vi "MyTestSimple.vi"() -> ()   [LabVIEW 2018]
uses:
  VisionLibrariesXimea/xiLib/xiLIB_64bit/xiLIB/xiCamLib/xiCam/PRM/PRM/PRM_v2.ctl
  VisionLibrariesXimea/xiLib/xiLIB_64bit/xiLIB/xiCamLib/xiLIB/Typedefs/xiLIB - PRM_Type.ctl
  D:/codes labview/VisionLibrariesXimea/xiLib/xiLIB_64bit/xiLIB/xiCamLib/API/x64/xiApi.NETX64.dll
  VisionLibrariesXimea/xiLib/xiLIB_64bit/xiLIB/xiCamLib/API/x64/xiApi.NETX64.dll
  <vilib>/Platform/TimedLoop/XDataNode/timing_clust.ctl
  <vilib>/Platform/TimedLoop/XDataNode/nitl_modes.ctl
  <vilib>/Platform/TimedLoop/XDataNode/wakeup.ctl
  System.Drawing
  VisionLibrariesXimea/xiLib/xiLIB_64bit/xiLIB/xiCamLib/xiLIB/xiLIB - GetPRM_INFO.vi
  VisionLibrariesXimea/xiLib/xiLIB_64bit/xiLIB/xiCamLib/xiCam/Methods/xiCam - GetParam_Int32.vi
  VisionLibrariesXimea/xiLib/xiLIB_64bit/xiLIB/xiCamLib/xiCam/Methods/xiCam - GetParam_Float.vi
  VisionLibrariesXimea/xiLib/xiLIB_64bit/xiLIB/xiCamLib/xiCam/Methods/xiCam - GetParam_String.vi
  <vilib>/platform/TimedLoop/XDataNode/XDataNode.xnode
  <vilib>/Platform/TimedLoop/XDataNode/XDNodeRunTimeDep.lvlib
panel:
  in  "Tab Control":T1(tab)
  in  "get float":T2
  out "output":variant
  out "Type":T3
  out "Desc.":string
  in  "start single":bool
  out "Waveform Graph 2":u8[](graph)
  out "Intensity Graph":u8[][](graph)
  in  "start loop acquire":bool
  out "Waveform Graph":u8[](graph)
  out "Numeric":i32
  out "Image":T4(plugin-control)
  in  "start NET":bool
  out "Numeric 2":i32
  in  "clear error":bool
  in  "dimension size":i32=16106496
  out "error out":errorcluster
  in  "stop":bool
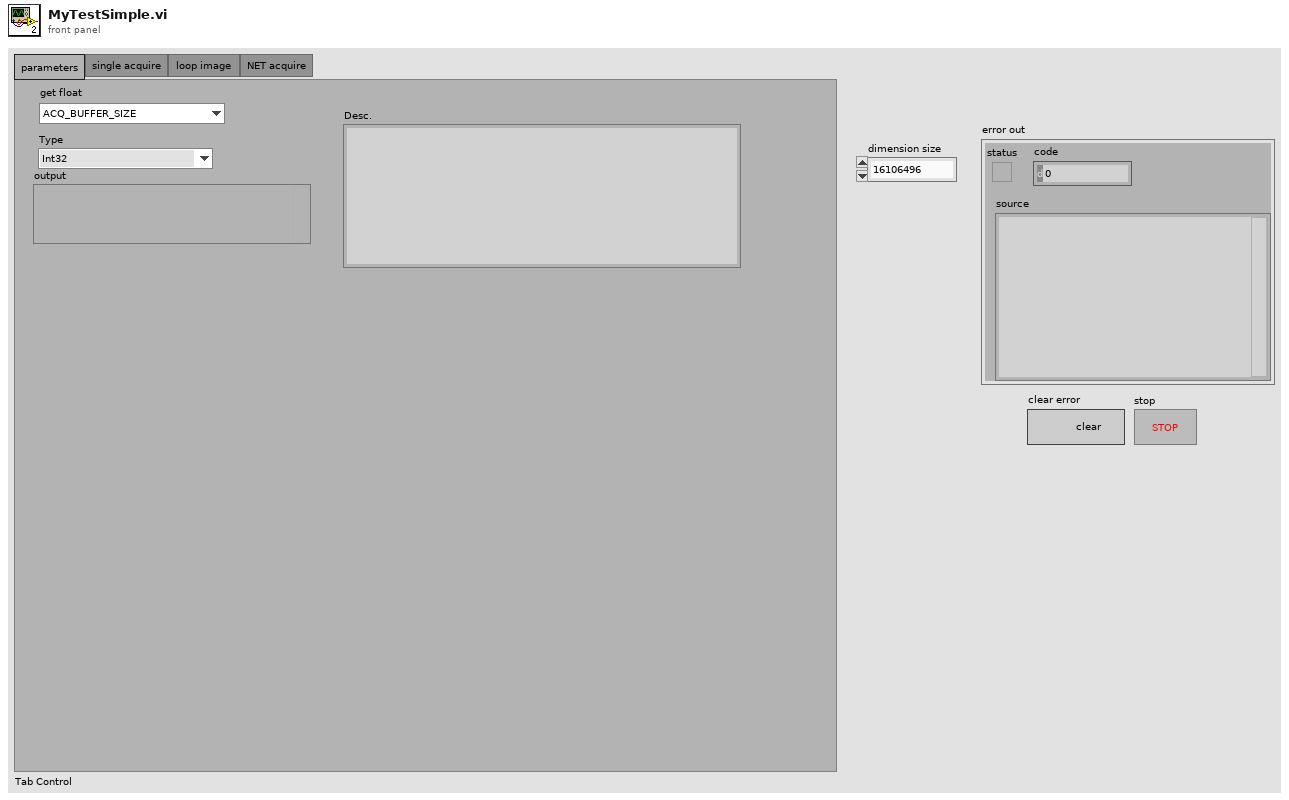
[diagram p1: front panel]
types:
  T1 = enum32{"parameters", "single acquire", "loop image ", "NET acquire"}
  T2 = typedef "PRM_v2.ctl" = enum16{"ACQ_BUFFER_SIZE", "ACQ_FRAME_BURST_COUNT", "ACQ_TIMING_MODE", "ACQ_TRANSPORT_BUFFER_SIZE", "AE_MAX_LIMIT", "AEAG", "AEAG_LEVEL", "API_VERSION", "AG_MAX_LIMIT", "APPLY_CMS", "AUTO_BANDWIDTH_CALCULATION", "AUTO_WB", "AVAILABLE_BANDWIDTH", "AVAILABLE_BANDWIDTH_MAX", "AVAILABLE_BANDWIDTH_MIN", "BPC", "BUFFER_POLICY", "BUFFERS_QUEUE_SIZE", "CC_MATRIX_00", "CC_MATRIX_01", "CC_MATRIX_02", "CC_MATRIX_03", "CC_MATRIX_10", "CC_MATRIX_11", "CC_MATRIX_12", "CC_MATRIX_13", "CC_MATRIX_20", "CC_MATRIX_21", "CC_MATRIX_22", "CC_MATRIX_23", "CC_MATRIX_30", "CC_MATRIX_31", "CC_MATRIX_32", "CC_MATRIX_33", "CHIP_TEMP", "CMS", "COLOR_FILTER_ARRAY", "COOLING", "DEBOUNCE_EN", "DEBOUNCE_POL", "DEBOUNCE_T0", "DEBOUNCE_T1", "DEBUG_LEVEL", "DEFAULT_CC_MATRIX", "DEVICE_INSTANCE_PATH", "DEVICE_MODEL_ID", "DEVICE_NAME", "DEVICE_SN", "DEVICE_TYPE", "DEVICE_USER_ID", "DOWNSAMPLING", "DOWNSAMPLING_MAX", "DOWNSAMPLING_MIN", "DOWNSAMPLING_TYPE", "DRV_VERSION", "EXP_PRIORITY", "EXPOSURE", "EXPOSURE_DIRECT_UPDATE", "EXPOSURE_MAX", "EXPOSURE_MIN", "FFS_FILE_NAME", "FPGA1_VERSION", "FRAMERATE", "FRAMERATE_MAX", "FRAMERATE_MIN", "FREE_FFS_SIZE", "GAIN", "GAIN_DIRECT_UPDATE", "GAIN_MAX", "GAIN_MIN", "GAMMAC", "GAMMAY", "GPI_LEVEL", "GPI_MODE", "GPI_SELECTOR", "GPI_SELECTOR_MAX", "GPI_SELECTOR_MIN", "GPO_MODE", "GPO_SELECTOR", "GPO_SELECTOR_MAX", "GPO_SELECTOR_MIN", "HDR", "HDR_T1", "HDR_T2", "HEIGHT", "HEIGHT_MAX", "HEIGHT_MIN", "HOUSE_TEMP", "IMAGE_DATA_FORMAT", "IMAGE_IS_COLOR", "INPUT_CMS_PROFILE", "IS_COOLED", "IS_DEVICE_EXIST", "KNEEPOINT1", "KNEEPOINT2", "LED_MODE", "LED_SELECTOR", "LED_SELECTOR_MAX", "LED_SELECTOR_MIN", "LIMIT_BANDWIDTH", "LIMIT_BANDWIDTH_MAX", "LIMIT_BANDWIDTH_MIN", "LUT_EN", "LUT_INDEX", "LUT_INDEX_MAX", "LUT_INDEX_MIN", "LUT_VALUE", "LUT_VALUE_MAX", "LUT_VALUE_MIN", "MANUAL_WB", "MCU1_VERSION", "MCU2_VERSION", "OFFSET_X", "OFFSET_X_MAX", "OFFSET_X_MIN", "OFFSET_Y", "OFFSET_Y_MAX", "OFFSET_Y_MIN", "OUTPUT_CMS_PROFILE", "OUTPUT_DATA_BIT_DEPTH", "OUTPUT_DATA_PACKING", "READ_FILE_FFS", "RECENT_FRAME", "SENSOR_DATA_BIT_DEPTH", "SENSOR_MODE", "SENSOR_TAPS", "SHARPNESS", "SHUTTER_TYPE", "TARGET_TEMP", "TRG_DELAY", "TRG_SELECTOR", "TRG_SOFTWARE", "TRG_SOURCE", "USED_FFS_SIZE", "WB_KB", "WB_KG", "WB_KR", "WIDTH", "WIDTH_MAX", "WIDTH_MIN", "WRITE_FILE_FFS", "ACQ_BUFFER_SIZE_UNIT", "ACQ_TRANSPORT_BUFFER_COMMIT", "AEAG_ROI_HEIGHT", "AEAG_ROI_OFFSET_X", "AEAG_ROU_OFFSET_Y", "AEAG_ROI_WIDTH", "API_CONTEXT_LIST", "BINNING_HORIZONTAL", "BINNING_SELECTOR", "BINNING_VERTICAL", "COLUMN_FPN_CORRECTION", "COUNTER_SELECTOR", "COUNTER_VALUE", "DECIMATION_HORIZONTAL", "DECIMATION_SELECTOR", "DECIMATION_VERTICAL", "DEVICE_ID", "DEVICE_LOCATION_PATH", "DEVICE_MANIFEST", "DEVICE_RESET", "DEVICE_SENS_SN", "EXPOSURE_BURST_COUNT", "FFS_ACCESS_KEY", "GAIN_SELECTOR", "HW_REVISION", "IMAGE_BLACK_LEVEL", "IMAGE_DATA_BIT_DEPTH", "IMAGE_DATA_FORMAT_RGB32_ALPHA", "IMAGE_PAYLOAD_SIZE", "LENS_APERTURE_VALUE", "LENS_FEATURE", "LENS_FEATURE_SELECTOR", "LENS_FOCAL_LENGTH", "LENS_FOCUS_DISTANCE", "LENS_FOCUS_MOVE", "LENS_FOCUS_MOVEMENT_VALUE", "LENS_MODE", "OUTPUT_DATA_PACKING_TYPE", "SENSOR_CLOCK_FREQ_HZ", "SENSOR_CLOCK_FREQ_INDEX", "SENSOR_FEATURE_SELECTOR", "SENSOR_FEATURE_VALUE", "SENSOR_OUTPUT_CHANNEL_COUNT", "TRANSPORT_PIXEL_FORMAT", "TS_RST_MODE", "TS_RST_SOURCE"}
  T3 = typedef "xiLIB - PRM_Type.ctl" = enum16{"Int32", "Float", "String", "DOWNSAMPLING_TYPE", "IMAGE_DATA_FORMAT", "BUFFER_POLICY", "TRG_SOURCE", "GPI", "GPO", "ACQ_TIMING_MODE", "BINNING_PATTERN", "BINNING_SELECTOR", "CMS_MODE", "COUNTER_SELECTOR", "DEBUG_LEVEL", "DECIMATION_PATTERN", "DECIMATION_SELECTOR", "GAIN_SELECTOR_TYPE", "LED_MODE", "LENS_FEATURE_SELECTOR", "LENS_MODE", "OUTPUT_DATA_PACKING_TYPE", "SENSOR_FEATURE_SELECTOR", "SHUTTER_TYPE", "TRG_SELECTOR", "TS_RST_MODE", "TS_RST_SOURCE"}
  T4 = typedef "IMAQ Image.ctl" = refnum<image>
  T5 = enum32{"Map Pixel Pointer", "Unmap Pixel Pointer", "Get Pixels Infos"}
  T6 = typedef "Image Type" = u32
  T7 = typedef "XDNodeRunTimeDep.lvlib/timing_clust.ctl" = cluster{"Expected End [f-1]":u64, "Actual End [f-1]":u64, "Finished Late? [f-1]":bool, "Expected End [i-1]":u64, "Actual End [i-1]":u64, "Finished Late? [i-1]":bool, "Expected Start [i]":u64, "Actual Start [i]":u64, "Expected Start [f]":u64, "Actual Start [f]":u64, "Source Name":string, "Structure Name":string, "Period":i64, "Deadline":i64, "Offset":i64, "Start":i64, "Priority":i32, "Timeout":i32, "Mode":T8, "Wakeup Reason":T9, "Error":errorcluster, "Source Type":string, "Secondary Source Type":string, "Global End Time":u64, "Global Start Time":u64, "Frame Duration":u64, "Iteration Duration":u64, "Assigned CPU":i32, "I/O Scan Engine Mode":u32}
  T8 = typedef "XDNodeRunTimeDep.lvlib/nitl_modes.ctl" = enum32{"No Change", "Process missed periods, maintain original phase", "Discard missed periods, maintain original phase", "Process missed periods, ignore original phase", "Discard missed periods, ignore original phase"}
  T9 = typedef "XDNodeRunTimeDep.lvlib/wakeup.ctl" = enum32{"Normal", "Aborted", "Asynchronous wakeup", "Timing source error", "Timed loop error", "Timeout"}
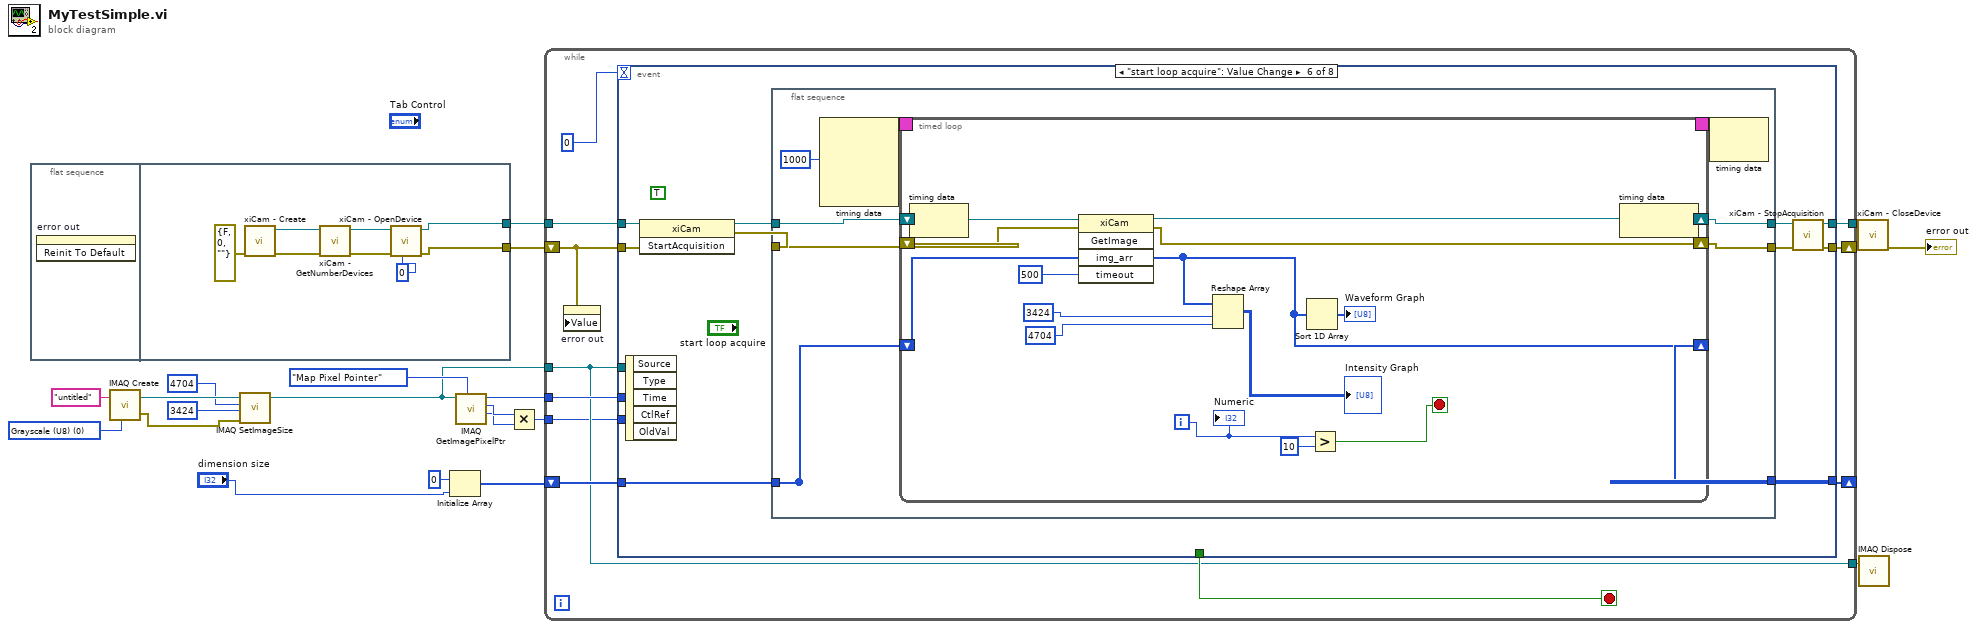
[diagram p0: block diagram]
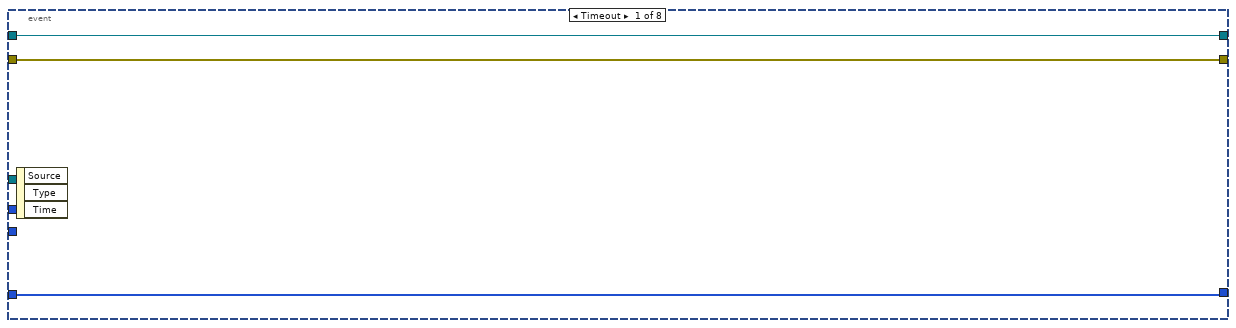
[diagram p2: hidden frame]
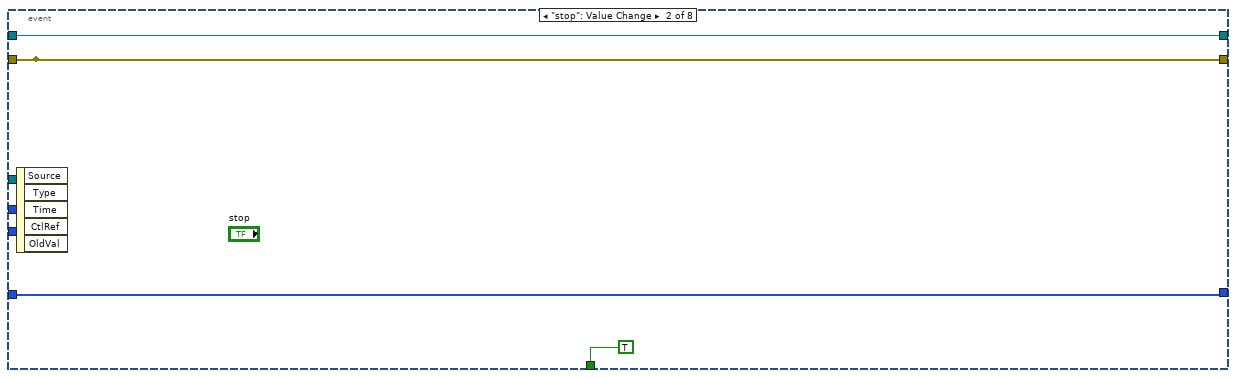
[diagram p3: hidden frame]
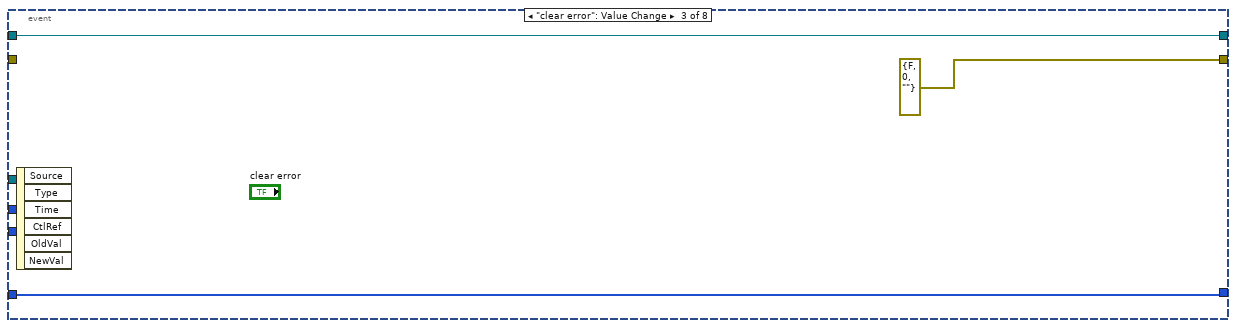
[diagram p4: hidden frame]
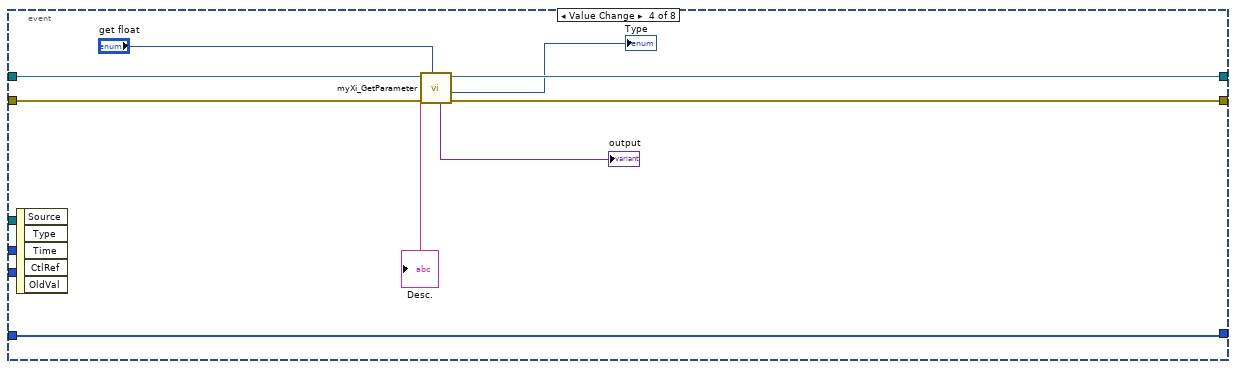
[diagram p5: hidden frame]
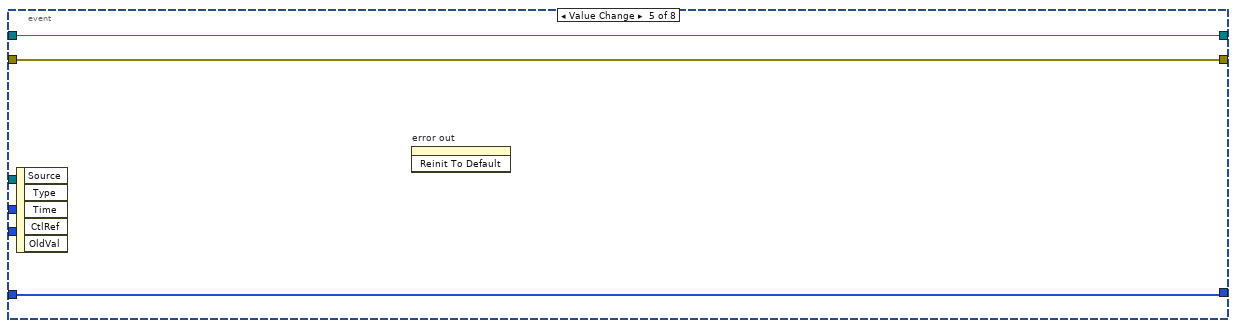
[diagram p6: hidden frame]
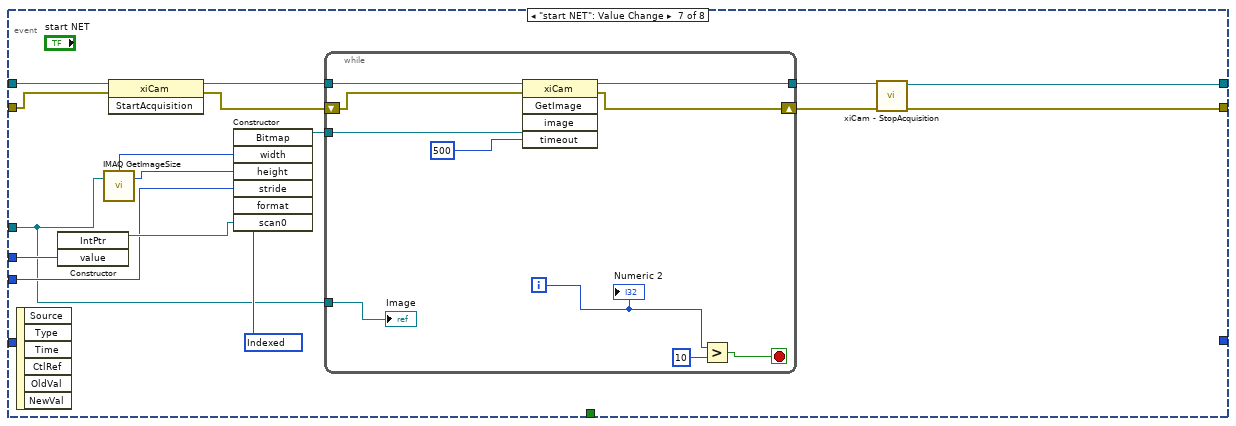
[diagram p7: hidden frame]
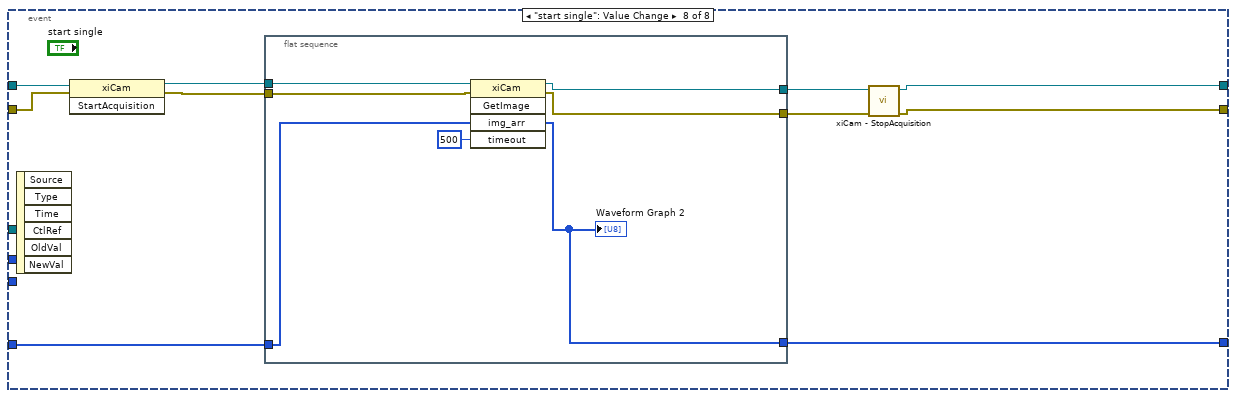
[diagram p8: hidden frame]
diagram:
  w12 = T6 0 items=["Grayscale (U8)", "Grayscale (I16)", "Grayscale (SGL)", "Complex (CSG)", "RGB (U32)", "HSL (U32)", "RGB (U64)", "Grayscale (U16)"] ("Image Type")
  n1 = flat-sequence {
    tunnel: [w23] -> w18
    tunnel: [w22] -> w17
    frame #0 {
      n2 = invoke on="error out" class="Clust (strict)" method="Reinit To Default"() -> ()  [unwired: 3 in, 3 out]
    }
    frame #1 {
      n3 = call "xiCam - Create.vi"("error in (no error)"=errorcluster {"status"=FALSE, "code"=0, "source"=""}) -> ("error out"=w27:errorcluster, "new xiCam"=w26:refnum<k24>)  [unwired: 9 in]
      n4 = call "xiCam - GetNumberDevices.vi"("error in (no error)"=w27, "xiCam In"=w26) -> ("error out"=w29:errorcluster, "xiCam Out"=w28:refnum<k24>)  [unwired: 7 in, 1 out]
      n5 = call "xiCam - OpenDevice.vi"("DevID"=0, "error in (no error)"=w29, "xiCam In"=w28) -> ("error out"=w22:errorcluster, "xiCam Out"=w23:refnum<k24>)  [unwired: 7 in]
    }
  }
  n6 = call "IMAQ Create"("Image Name"="untitled", "Image Type"=w12) -> ("New Image"=w11:T4, "error out"=w8:errorcluster)  [unwired: 3 in]
  n7 = call "IMAQ SetImageSize"("error in (no error)"=w8, "Y Resolution"=3424 ("height"), "X Resolution"=4704, "Image"=w11) -> ("Image Out"=w5:T4)  [unwired: 1 in, 1 out]
  n8 = Initialize Array(u8 0 ("element"), "dimension size") -> (w14:u8[])
  n9 = call "IMAQ GetImagePixelPtr"("Function"=T5."Map Pixel Pointer", "Image"=w5) -> ("Pixel Size (Bytes)"=w2:i32, "LineWidth(Pixels)"=w3:i32, "Pixel Pointer out"=w6:u64)  [unwired: 4 in, 3 out]
  n10 = Multiply(x=w3, y=w2) -> (x*y=w1:i32)
  n11 = while {
    tunnel: [w39] -> w21
    tunnel: w18 -> [w40]
    shift-right: [w37] -> w19
    shift-left: w17 -> [w36]
    shift-right: [w33] -> _
    shift-left: w14 -> [w34]
    tunnel: w6 -> [w32]
    tunnel: w5 -> [w31]
    tunnel: [w31] -> w4
    tunnel: w1 -> [w30]
    stop <- w38 stop-if-true
    n12 = property on="error out" class="Clust (strict)"("Value"=w36) -> ()  [unwired: 2 in, 2 out]
    n13 = event shown="[5] \"start loop acquire\": Value Change" {
      selector: _ -> [_ _ _ _ _ _ _ _]
      dyn-events: _ -> [_ _ _ _ _ _ _ _]
      timeout: 0 -> [_ _ _ _ _ _ _ _]
      tunnel: w40 -> [w43 w46 w50 w57 w62 w71 w106 w137]
      tunnel: [w43 w46 w50 w54 w62 w72 w114 w136] -> w39
      tunnel: w36 -> [w42 w45 _ w59 w61 w69 w104 w128]
      tunnel: [w42 w45 errorcluster {"status"=FALSE, "code"=0, "source"=""} ("error out") w58 w61 w63 w116 w135] -> w37
      tunnel: [_ TRUE ("stop") _ _ _ _ _ _] -> w38
      tunnel: [_ w45 _ _ _ _ _ _] -> _
      tunnel: w34 -> [w41 w44 w48 w51 w60 w66 _ w133]
      tunnel: [w41 w44 w48 w51 w60 w65 _ w132] -> w33
      tunnel: w32 -> [_ _ _ _ _ _ w112 _]
      tunnel: w31 -> [_ _ _ _ _ _ w102 _]
      tunnel: w30 -> [_ _ _ _ _ _ w107 _]
      event Timeout {
        n14 = event-data() -> ()  [unwired: 1 in, 3 out]
      }
      event "stop": Value Change {
        n15 = event-data() -> ()  [unwired: 1 in, 5 out]
      }
      event "clear error": Value Change {
        n16 = event-data() -> ()  [unwired: 1 in, 6 out]
      }
      event Value Change {
        n17 = event-data() -> ()  [unwired: 1 in, 5 out]
        n18 = call "myXi_GetParameter.vi"("input PRM"="get float", "error in"=w59, "xiCam IN"=w57) -> ("error out"=w58:errorcluster, "Type"=→"Type":T3, "xiCam Out"=w54:refnum<k24>, "output"=→"output":variant, "Desc."=→"Desc.":string)  [unwired: 3 in, 1 out]
      }
      event "error out.status": Value Change {
        n19 = event-data() -> ()  [unwired: 1 in, 5 out]
        n20 = invoke on="error out" class="Clust (strict)" method="Reinit To Default"() -> ()  [unwired: 3 in, 3 out]
      }
      event "start loop acquire": Value Change {
        (unwired) TRUE ("Boolean")
        n21 = event-data() -> ()  [unwired: 1 in, 5 out]
        n22 = invoke class="xiCam" method="StartAcquisition"(reference=w71, error in=w69) -> (reference out=w70:refnum<k24>, error out=w64:errorcluster)  [unwired: 1 in, 1 out]
        n23 = flat-sequence {
          tunnel: w64 -> [w79]
          tunnel: w70 -> [w81]
          tunnel: [w80] -> w68
          tunnel: [w78] -> w67
          tunnel: w66 -> [w77]
          tunnel: [w76] -> w65
          tunnel: [w77] -> _
          frame #0 {
            n24 = node-c288(i64 1000 ("Period")) -> (w75:T7)  [unwired: 3 in]
            n25 = timed-loop {
              shift-right: [w95] -> w80
              shift-left: w81 -> [w86]
              shift-right: [w92] -> w78
              shift-left: w79 -> [w93]
              shift-right: [w85] -> w76
              shift-left: w77 -> [w91]
              timing: w75 -> [_]
              timing-out: [_] -> w74
              i -> [w89]
              stop <- w87 stop-if-true
              n26 = node-c288() -> ()  [unwired: 1 in, 1 out]
              n27 = invoke class="xiCam" method="GetImage"(reference=w86, error in=w93, "img_arr"=w91, "timeout"=500) -> (reference out=w95:refnum<k24>, error out=w92:errorcluster, "img_arr"=w85:u8[])  [unwired: 1 in, 2 out]
              n28 = Reshape Array(w85, 3424 ("height"), 4704 ("X Resolution")) -> (→"Intensity Graph":u8[][])
              n29 = Sort 1D Array(array=w85) -> (sorted array=→"Waveform Graph":u8[])
              n30 = Greater?(x=w89, y=10) -> (0:w87:bool)
              n31 = node-c288() -> ()  [unwired: 1 in, 1 out]
              "Numeric" <- w89
            }
            n32 = node-c288(w74) -> ()  [unwired: 1 out]
          }
        }
        n33 = call "xiCam - StopAcquisition.vi"("error in (no error)"=w67, "xiCam In"=w68) -> ("error out"=w63:errorcluster, "xiCam Out"=w72:refnum<k24>)  [unwired: 8 in]
      }
      event "start NET": Value Change {
        w108 = 65536 items=["DontCare, Undefined"=0, "Max"=15, "Indexed"=65536, "Gdi"=131072, "Format16bppRgb555"=135173, "Format16bppRgb565"=135174, "Format24bppRgb"=137224, "Format32bppRgb"=139273, "Format1bppIndexed"=196865, "Format4bppIndexed"=197634, "Format8bppIndexed"=198659, "Alpha"=262144, "Format16bppArgb1555"=397319, "PAlpha"=524288, "Format32bppPArgb"=925707, "Extended"=1048576, "Format16bppGrayScale"=1052676, "Format48bppRgb"=1060876, "Format64bppPArgb"=1851406, "Canonical"=2097152, "Format32bppArgb"=2498570, "Format64bppArgb"=3424269] ("format")
        n34 = event-data() -> ()  [unwired: 1 in, 6 out]
        n35 = constructor class="IntPtr"("value"=w112) -> (reference out=w111:refnum<k24>)  [unwired: 3 in, 3 out]
        n36 = call "IMAQ GetImageSize"("Image"=w102) -> ("Y Resolution"=w109:i32, "X Resolution"=w110:i32)  [unwired: 1 in, 3 out]
        n37 = invoke class="xiCam" method="StartAcquisition"(reference=w106, error in=w104) -> (reference out=w105:refnum<k24>, error out=w103:errorcluster)  [unwired: 1 in, 1 out]
        n38 = constructor class="Bitmap"("width"=w110, "height"=w109, "stride"=w107, "format"=w108, "scan0"=w111) -> (reference out=w113:refnum<k24>)  [unwired: 3 in, 7 out]
        n39 = while {
          tunnel: w105 -> [w127]
          tunnel: [w126] -> w115
          shift-right: [w125] -> w117
          shift-left: w103 -> [w120]
          tunnel: w113 -> [w121]
          tunnel: w102 -> [w118]
          i -> [w122]
          stop <- w123 stop-if-true
          n40 = invoke class="xiCam" method="GetImage"(reference=w127, error in=w120, "image"=w121, "timeout"=500) -> (reference out=w126:refnum<k24>, error out=w125:errorcluster)  [unwired: 1 in, 3 out]
          n41 = Greater?(x=w122, y=10) -> (0:w123:bool)
          "Numeric 2" <- w122
          "Image" <- w118
        }
        n42 = call "xiCam - StopAcquisition.vi"("error in (no error)"=w117, "xiCam In"=w115) -> ("error out"=w116:errorcluster, "xiCam Out"=w114:refnum<k24>)  [unwired: 8 in]
      }
      event "start single": Value Change {
        n43 = event-data() -> ()  [unwired: 1 in, 6 out]
        n44 = invoke class="xiCam" method="StartAcquisition"(reference=w137, error in=w128) -> (reference out=w134:refnum<k24>, error out=w129:errorcluster)  [unwired: 1 in, 1 out]
        n45 = flat-sequence {
          tunnel: w134 -> [w144]
          tunnel: w133 -> [w143]
          tunnel: [w141] -> w132
          tunnel: [w140] -> w131
          tunnel: [w139] -> w130
          tunnel: w129 -> [w138]
          frame #0 {
            n46 = invoke class="xiCam" method="GetImage"(reference=w144, error in=w138, "img_arr"=w143, "timeout"=500) -> (reference out=w140:refnum<k24>, error out=w139:errorcluster, "img_arr"=w141:u8[])  [unwired: 1 in, 2 out]
            "Waveform Graph 2" <- w141
          }
        }
        n47 = call "xiCam - StopAcquisition.vi"("error in (no error)"=w130, "xiCam In"=w131) -> ("error out"=w135:errorcluster, "xiCam Out"=w136:refnum<k24>)  [unwired: 8 in]
      }
    }
  }
  n48 = call "xiCam - CloseDevice.vi"("error in (no error)"=w19, "xiCam In"=w21) -> ("error out"=→"error out":errorcluster)  [unwired: 9 in]
  n49 = call "IMAQ Dispose"("Image"=w4) -> ()  [unwired: 5 in, 1 out]
